vi "Process Peek Window Scroll.vi"(4 "Inserted Window":T1, 5 "SubPanel":refnum<vi>, 6 "error in (no error)":errorcluster, 9 "Process Peek Window Scroll Argument":T2) -> (0 "error out":errorcluster)   [LabVIEW 2020, in "Peek Window.lvlib"]
doc: "Processes the Mouse Scroll on the sub panel where the VI Block Diagram Window is inserted. And update the Block Diagram origin according to simulate the normal scroll operations on the Block Diagram.\n\nWhen VI Front Panel Window is inserted into a Subpanel, the scrolling operations are implicitly available.\nSo only for the inserted Block Diagram Windows, we want to simulate the Scroll."
uses:
  Peek Window.lvlib
  Scroll Data.ctl
  <vilib>/Utility/miscctls.llb/LVPoint32TypeDef.ctl
  <vilib>/Utility/traverseref.llb/TRef TravTarget.ctl
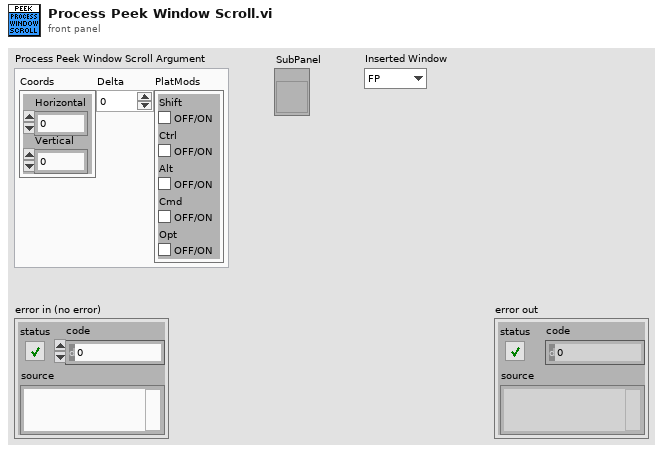
[diagram p1: front panel]
types:
  T1 = typedef "TRef TravTarget.ctl" = enum16{"FP", "BD", "Other"}
  T2 = typedef "Peek Window.lvlib/Scroll Data.ctl" = cluster{"Coords":T3, "Delta":i32, "PlatMods":cluster{"Shift":bool, "Ctrl":bool, "Alt":bool, "Cmd":bool, "Opt":bool}}
  T3 = typedef "LVPoint32TypeDef.ctl" = cluster{"Horizontal":i32, "Vertical":i32}
  T4 = typedef "LVRectTypeDef.ctl" = cluster{"Left":i16, "Top":i16, "Right":i16, "Bottom":i16}
  T5 = typedef "LVPointTypeDef.ctl" = cluster{"Horizontal":i16, "Vertical":i16}
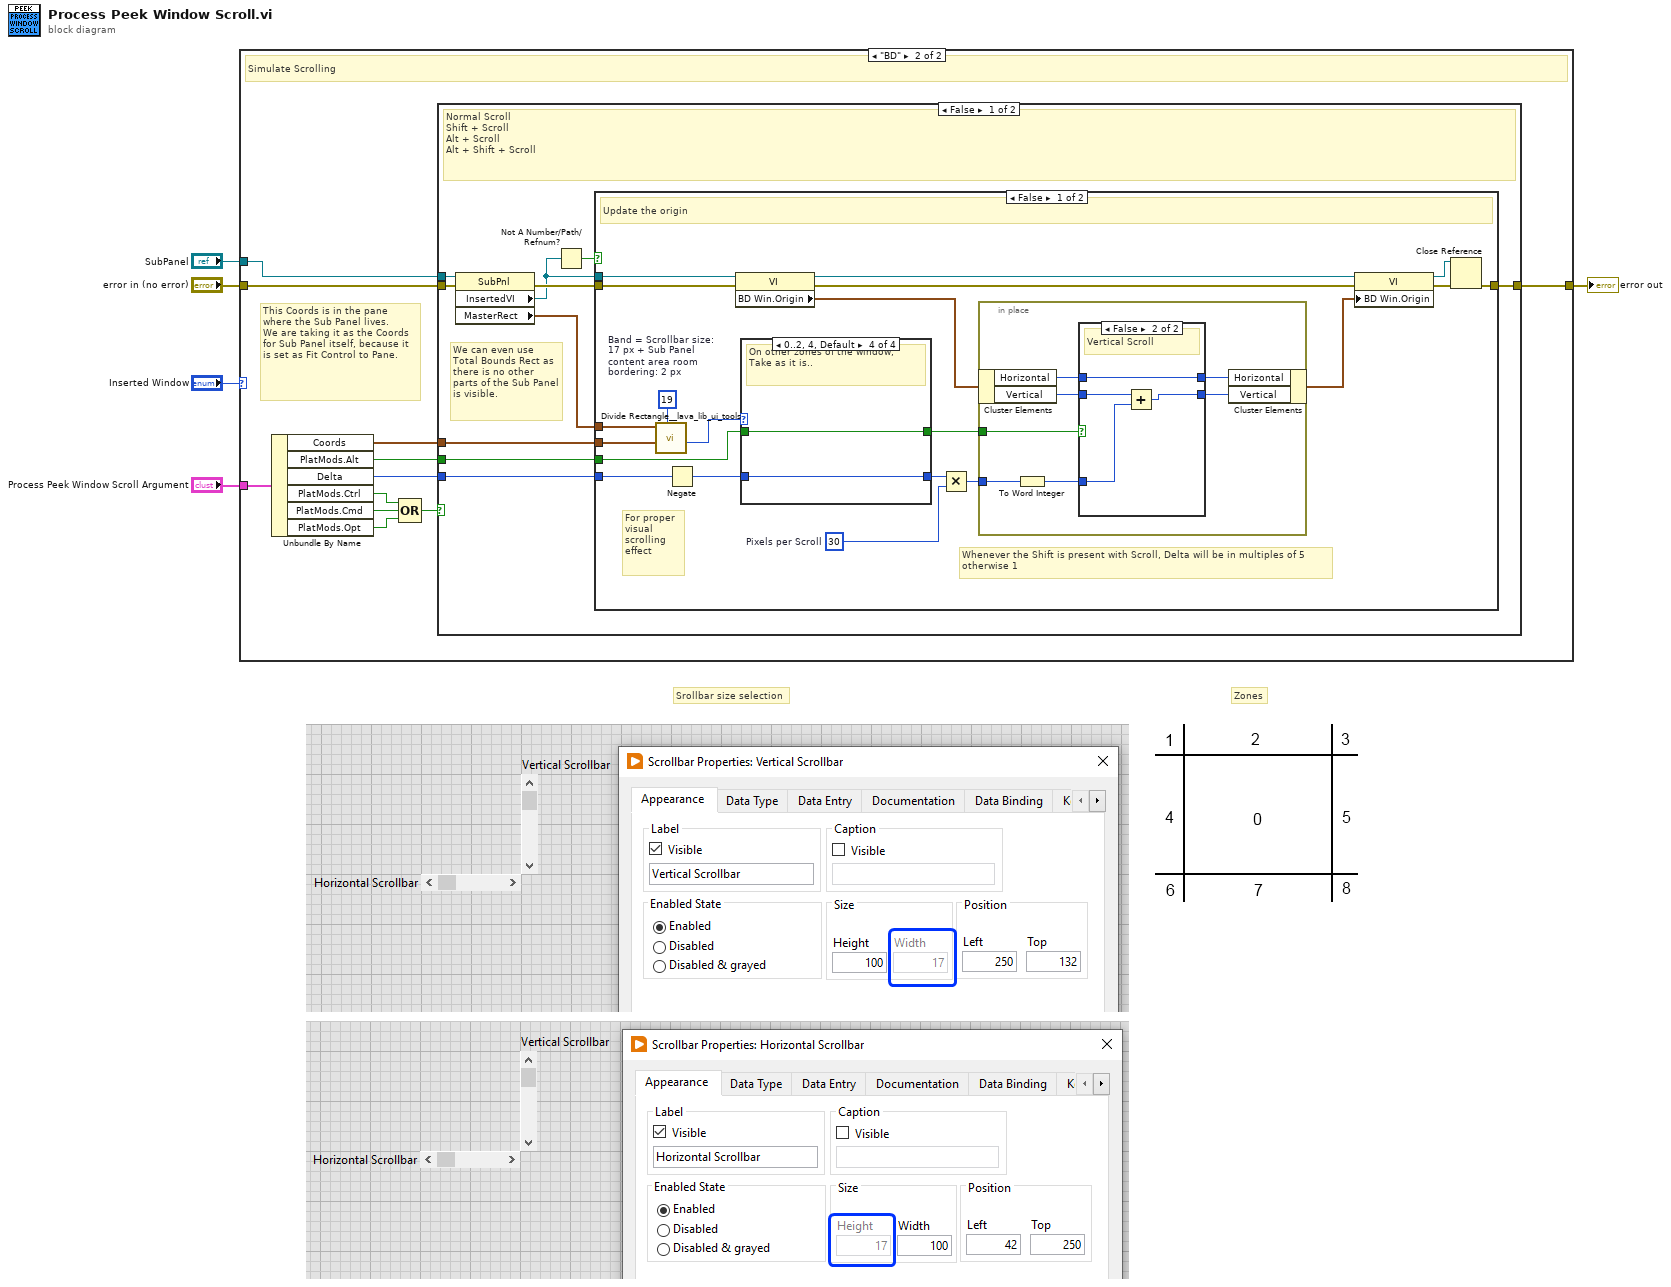
[diagram p0: block diagram]
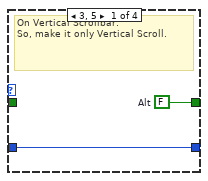
[diagram p3: hidden frame]
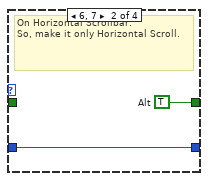
[diagram p4: hidden frame]
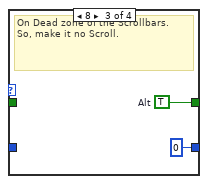
[diagram p5: hidden frame]
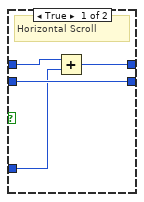
[diagram p6: hidden frame]
diagram:
  # "Srollbar size selection"
  # "Zones"
  n1 = case shown="\"BD\"" "Inserted Window" {
    tunnel: "Process Peek Window Scroll Argument" -> [_ w17]
    tunnel: "error in (no error)" -> [w6 w16]
    tunnel: "SubPanel" -> [_ w15]
    tunnel: [w6 w14] -> w2
    frame "FP", Default {
      # "When VI Front Panel Window is inserted into a Subpanel, the scrolling operations are implicitly available."
    }
    frame "BD" {
      # "This Coords is in the pane where the Sub Panel lives.\nWe are taking it as the Coords for Sub Panel itself, because it is set as Fit Control to Pane."
      # "Simulate Scrolling"
      n2 = Unbundle By Name(w17) -> ("Coords"=w9:T3, "PlatMods.Alt"=w7:bool, "Delta"=w8:i32, "PlatMods.Ctrl"=w13:bool, "PlatMods.Cmd"=w12:bool, "PlatMods.Opt"=w11:bool)
      n3 = Compound Arithmetic op=OR(w13, w12, w11) -> (w10:bool)
      n4 = case shown="False" w10 {
        tunnel: w16 -> [w27 w72]
        tunnel: w15 -> [w26 _]
        tunnel: [w24 w72] -> w14
        tunnel: w8 -> [w23 _]
        tunnel: w7 -> [w22 _]
        tunnel: w9 -> [w19 _]
        frame False {
          # "We can even use Total Bounds Rect as there is no other parts of the Sub Panel is visible."
          # "Normal Scroll\nShift + Scroll\nAlt + Scroll\nAlt + Shift + Scroll"
          n5 = property class="SubPnl"(reference=w26, error in=w27) -> (error out=w25:errorcluster, "InsertedVI"=w21:refnum<vi>, "MasterRect"=w18:T4)  [unwired: 1 out]
          n6 = Not A Number/Path/Refnum?(number/path/refnum=w21) -> (NaN/Path/Refnum?=w20:bool)
          n7 = case shown="False" w20 {
            tunnel: w25 -> [w47 w71]
            tunnel: w21 -> [w45 _]
            tunnel: [w29 w71] -> w24
            tunnel: w23 -> [w40 _]
            tunnel: w22 -> [w33 _]
            tunnel: w19 -> [w37 _]
            tunnel: w18 -> [w36 _]
            frame False {
              w35 = i16 19  # Band = Scrollbar size: 17 px + Sub Panel content area room bordering: 2 px
              w38 = 30  # Pixels per Scroll
              # "For proper visual scrolling effect"
              # "Whenever the Shift is present with Scroll, Delta will be in multiples of 5\notherwise 1"
              # "Update the origin"
              n8 = call <vilib>:"Divide Rectangle__lava_lib_ui_tools.vi"("Band (50)"=w35, "Coords"=w37, "Rectangle"=w36) -> ("Zone"=w34:i32)  [unwired: 7 in, 1 out]
              n9 = Negate(x=w40) -> (-x=w31:i32)
              n10 = property class="VI"(reference=w45, error in=w47) -> (reference out=w43:refnum<vi>, error out=w46:errorcluster, "BD Win.Origin"=w42:T5)
              n11 = case shown="0..2, 4, Default" w34 {
                tunnel: w33 -> [_ _ _ w55]
                tunnel: [w49 w51 w53 w55] -> w32
                tunnel: w31 -> [w48 w50 _ w54]
                tunnel: [w48 w50 0 w54] -> w30
                frame 3, 5 {
                  w49 = FALSE  # Alt
                  # "On Vertical Scrollbar.\nSo, make it only Vertical Scroll."
                }
                frame 6, 7 {
                  w51 = TRUE  # Alt
                  # "On Horizontal Scrollbar.\nSo, make it only Horizontal Scroll."
                }
                frame 8 {
                  w53 = TRUE  # Alt
                  # "On Dead zone of the Scrollbars.\nSo, make it no Scroll."
                }
                frame 0..2, 4, Default {
                  # "On other zones of the window,\nTake as it is.."
                }
              }
              n12 = Multiply(x=w30, y=w38) -> (x*y=w39:i32)
              n13 = in-place {
                in-place-border: w39 -> [w62]
                in-place-border: w32 -> [w61]
                n14 = in-place-cluster #1(w42) -> ("Horizontal"=w60:i16, "Vertical"=w58:i16)
                n15 = To Word Integer(number=w62) -> (16bit integer=w56:i16)
                n16 = case shown="False" w61 {
                  tunnel: w56 -> [w63 w67]
                  tunnel: w60 -> [w65 w69]
                  tunnel: [w66 w68] -> w59
                  tunnel: w58 -> [w66 w70]
                  tunnel: [w64 w69] -> w57
                  frame True {
                    # "Horizontal Scroll"
                    n17 = Add(x=w65, y=w63) -> (x+y=w64:i16)
                  }
                  frame False {
                    # "Vertical Scroll"
                    n18 = Add(x=w70, y=w67) -> (x+y=w68:i16)
                  }
                }
                n19 = in-place-cluster #1("Horizontal"=w57, "Vertical"=w59) -> (w41:T5)
              }
              n20 = property class="VI"(reference=w43, error in=w46, "BD Win.Origin"=w41) -> (reference out=w28:refnum<vi>, error out=w44:errorcluster)
              n21 = Close Reference(reference=w28, error in (no error)=w44) -> (error out=w29:errorcluster)
            }
            frame True {
              # "No VI BD have been inserted so far"
            }
          }
        }
        frame True {
          # "These PlatMods are used to interact with the Block Diagram"
        }
      }
    }
  }
  "error out" <- w2
